vi "CThread Set Selector Terminal.vi"   [LabVIEW 2012, in "CThread.lvlib"]
uses:
  CThread.lvlib
  XNodes/terminalnode/CThread VI Terminal Node.xnode
  Base/CThread Base - Set Selector Terminal.vi
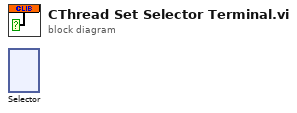
[diagram p0: block diagram]
diagram:
  n1 = xnode "Selector"() -> ()  [unwired: 2 in, 1 out]
